vi "analyze.vi"(7 "worker ID (0)":u32, 9 "error in":errorcluster, 10 "duration (s)":dbl, 11 "relative seconds":dbl[](array[numeric])) -> (1 "error out":errorcluster, 2 "metadata":T1, 3 "data":dbl[][](array[numeric]))   [LabVIEW 2020]
uses:
  metadata.ctl
  <vilib>/Analysis/baseanly.llb/Mean (DBL).vi
  <vilib>/Analysis/NI_AALBase.lvlib
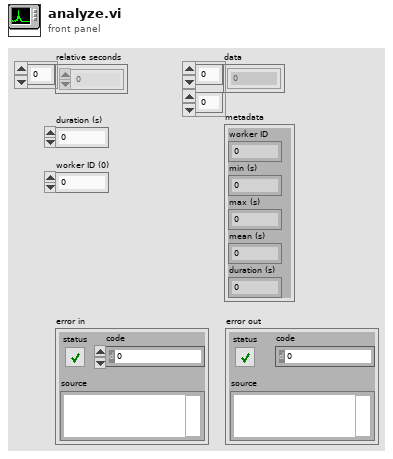
[diagram p1: front panel]
types:
  T1 = typedef "metadata.ctl" = cluster{"worker ID":u32, "min (s)":dbl, "max (s)":dbl, "mean (s)":dbl, "duration (s)":dbl}
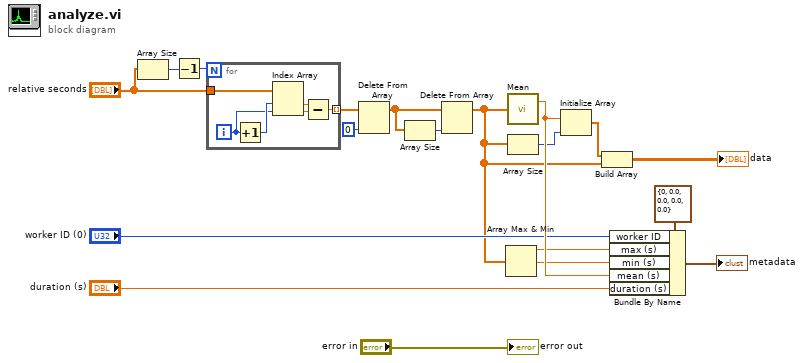
[diagram p0: block diagram]
diagram:
  n1 = Array Size(array="relative seconds") -> (size(s)=w10:i32)
  n2 = Decrement(x=w10) -> (x-1=w11:i32)
  n3 = for {
    N: w11 -> [_]
    tunnel: "relative seconds" -> [w24]
    tunnel: [w20] -> w5 mode=indexing
    i -> [w23]
    n4 = Increment(x=w23) -> (x+1=w25:i32)
    n5 = Index Array(array=w24, index #1=w25, index #2=w23) -> (element #1=w21:dbl, element #2=w22:dbl)
    n6 = Subtract(x=w21, y=w22) -> (x-y=w20:dbl)
  }
  n7 = Delete From Array(array=w5, index=0) -> (array with subset deleted=w1:dbl[])  [unwired: 1 in, 1 out]
  n8 = Array Size(array=w1) -> (size(s)=w2:i32)
  n9 = Delete From Array(array=w1, index=w2) -> (array with subset deleted=w4:dbl[])  [unwired: 1 in, 1 out]
  n10 = Array Max & Min(array=w4) -> (max value=w15:dbl, min value=w16:dbl)  [unwired: 2 out]
  n11 = call-poly <vilib>:"Mean.vi"("X"=w4) -> ("mean"=w17:dbl)  [unwired: 1 out]
  n12 = Array Size(array=w4) -> (size(s)=w12:i32)
  n13 = Initialize Array(w17, w12) -> (w7:dbl[])
  n14 = Build Array(w7, w4) -> (→"data":dbl[][])
  n15 = Bundle By Name(cluster=T1 {"worker ID"=0, "min (s)"=0.0, "max (s)"=0.0, "mean (s)"=0.0, "duration (s)"=0.0} ("Results"), "worker ID"="worker ID (0)", "max (s)"=w15, "min (s)"=w16, "mean (s)"=w17, "duration (s)"="duration (s)") -> (→"metadata":T1)
  "error out" <- "error in"
